vi "Defer Panel Updates.vi"(8 "error in (no error)":errorcluster, 10 "Defer Panel Updates":bool, 11 "PluginGUI in":refnum<class "PluginGUI.lvclass">) -> (0 "error out":errorcluster, 3 "PluginGUI out":refnum<class "PluginGUI.lvclass">)   [LabVIEW 2020, in "VolatusGUI.lvlib" / "PluginGUI.lvclass"]
uses:
  PluginGUI.lvclass
  PluginGUI.lvclass/PluginGUI.ctl
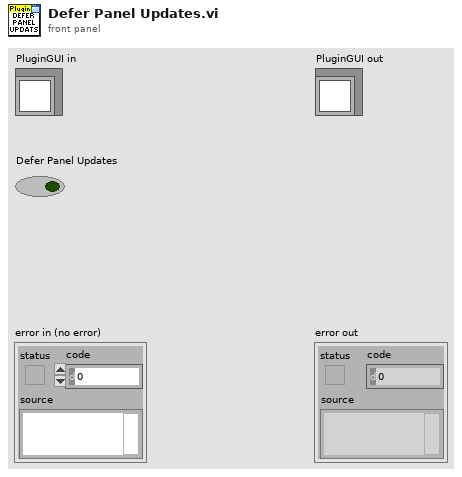
[diagram p1: front panel]
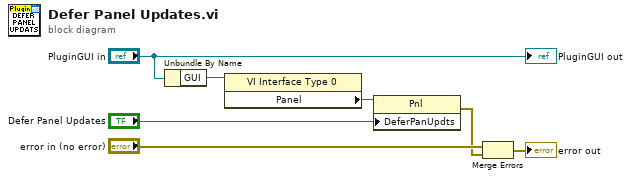
[diagram p0: block diagram]
diagram:
  n1 = Unbundle By Name("PluginGUI in") -> ("GUI"=w5:refnum<vi>)
  n2 = property class="VI Interface Type 0"(reference=w5) -> ("Panel"=w4:refnum<vi>)  [unwired: 1 in, 2 out]
  n3 = property class="Pnl"(reference=w4, "DeferPanUpdts"="Defer Panel Updates") -> (error out=w1:errorcluster)  [unwired: 1 in, 1 out]
  n4 = Merge Errors("error in (no error)", w1) -> (→"error out":errorcluster)
  "PluginGUI out" <- "PluginGUI in"
